vi "子VI-查看某框-不显示界面.vi"(0 "框号":dbl format="%#_13g", 1 "框组":T3(array[cluster]), 2 "计入缺陷的Z值阈值":i32 caption="值", 3 "临界Z值":i32, 4 "计入缺陷的面积阈值":i32, 5 "临界面积百分比值":dbl, 6 "图像Y向分辨率（mm/像素）":dbl, 7 "缺陷灰度阈值":dbl caption="值", 8 "?":T2(plugin-control), 9 "部位信息":string[](array[string])=["", "34.500000", "32.500000", "1121", "34", "54.955926", "分层类", "不合格", ""], 10 "判定为筋条的长宽比阈值":i32, 11 "图像X向分辨率（mm/像素）":dbl) -> (20 "全部检测结果":string[][](table), 25 "flag标记簇":cluster{"框号":dbl, "数值":i32})   [LabVIEW 2018]
uses:
  <vilib>/vision/NI_Vision_Development_Module.lvlib
panel:
  out "中心Y":dbl
  out "中心X":dbl
  in  "Tab Control":T1
  out "Threshold Image":T2(plugin-control)
  out "分层缺陷个数":i32
  out "合格？ 弥散类":string="fencengThreshold"
  out "合格？分层类":string="fencengThreshold"
  out "面积 (pixels)":i32
  in  "格式字符串 2":string="%f"
  in  "分隔符（'\\'代码显示）":string="\t"
  out "分层测量结果":i16[][](array[numeric])
  # "所选区域信息"
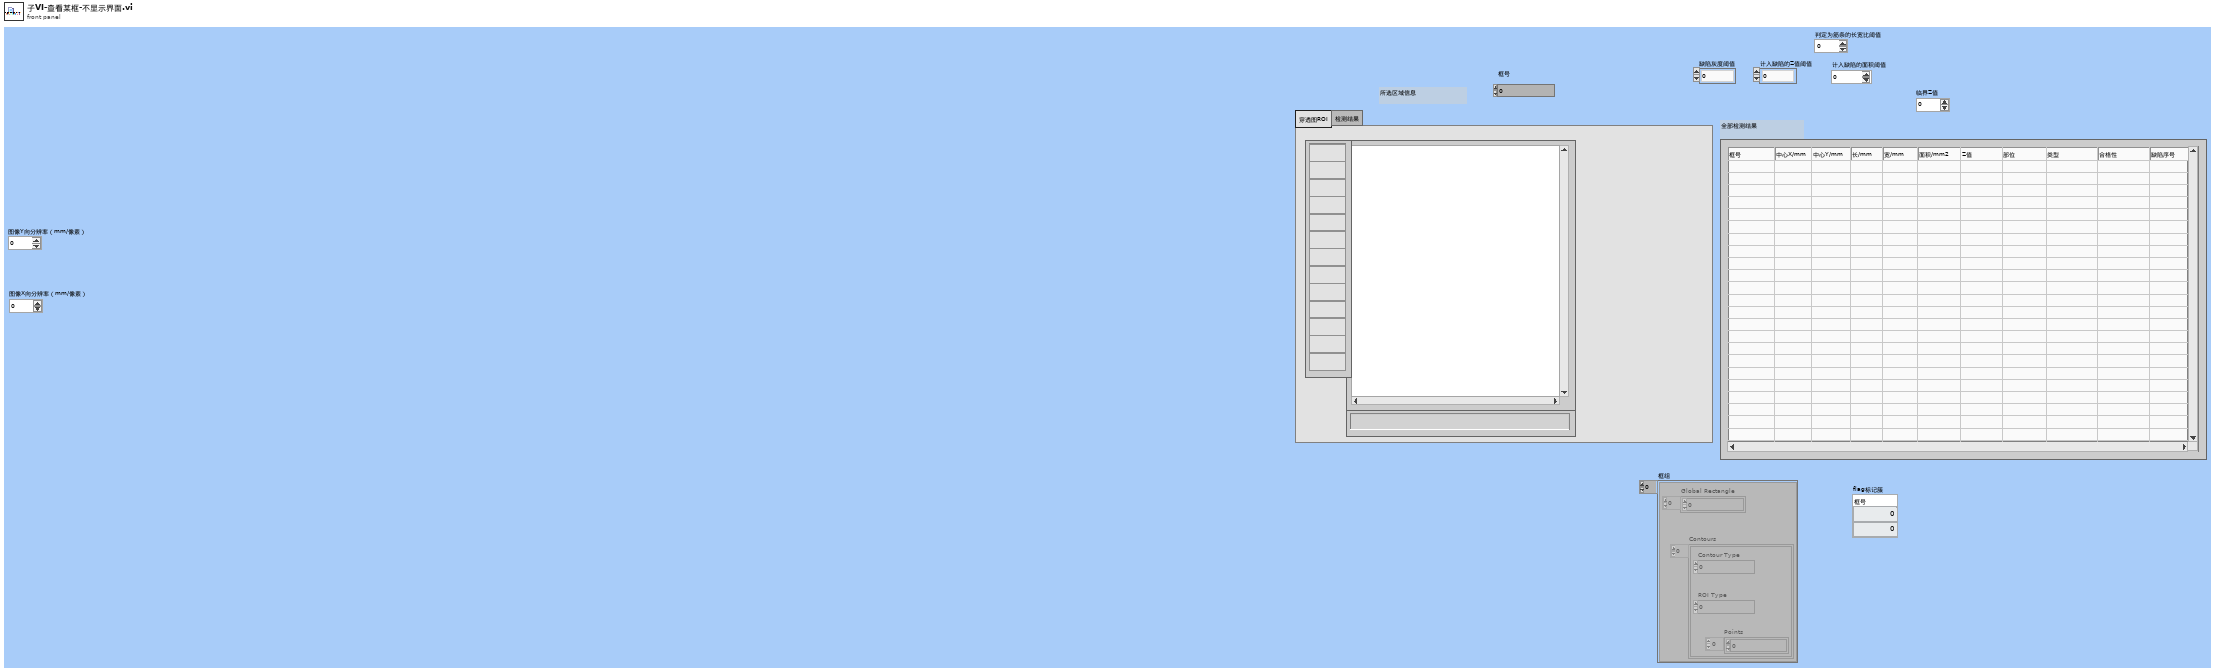
[diagram p1: front panel]
types:
  T1 = typedef "控件2.ctl" = enum32{"穿透图ROI", "检测结果"}
  T2 = typedef "IMAQ Image.ctl" = refnum<image>
  T3 = cluster{"Global Rectangle":i32[], "Contours":cluster{"Contour Type":u32, "ROI Type":u32, "Points":i32[]}[]}[]
  T4 = typedef "Image Type" = u32
  T5 = cluster{"Global Rectangle":i32[], "Contours":cluster{"Contour Type":u32, "ROI Type":u32, "Points":i32[]}[]}
  T6 = cluster{"Desired Font (Application)":enum16{"User-specified Font", "Application Font", "System Font", "Dialog Font"}, "[User-specified Font]":cluster{"Font Name":string, "Size":i16, "Strikeout?":bool, "Italic?":bool, "Underline?":bool, "Outline?":bool, "Shadow?":bool, "Bold?":bool, "Rotation Angle":dbl}, "Horizontal Alignment":i16, "Vertical Alignment":i16}
  T7 = cluster{"histogram":u32[], "Minimal Value":sgl, "Maximal Value":sgl, "Starting Value":sgl, "Interval Width":sgl, "Mean Value":sgl, "Standard  Variation":sgl, "Area (pixels)":i32}
  T8 = typedef "Particle Parameters" = i32
  T9 = cluster{"Area":dbl, "Number of Holes":dbl, "Bounding Rect":cluster{"Left":dbl, "Top":dbl, "Right":dbl, "Bottom":dbl}, "Center of Mass":cluster{"X":dbl, "Y":dbl}, "Orientation":dbl, "Dimensions":cluster{"Width":dbl, "Height":dbl}}[]
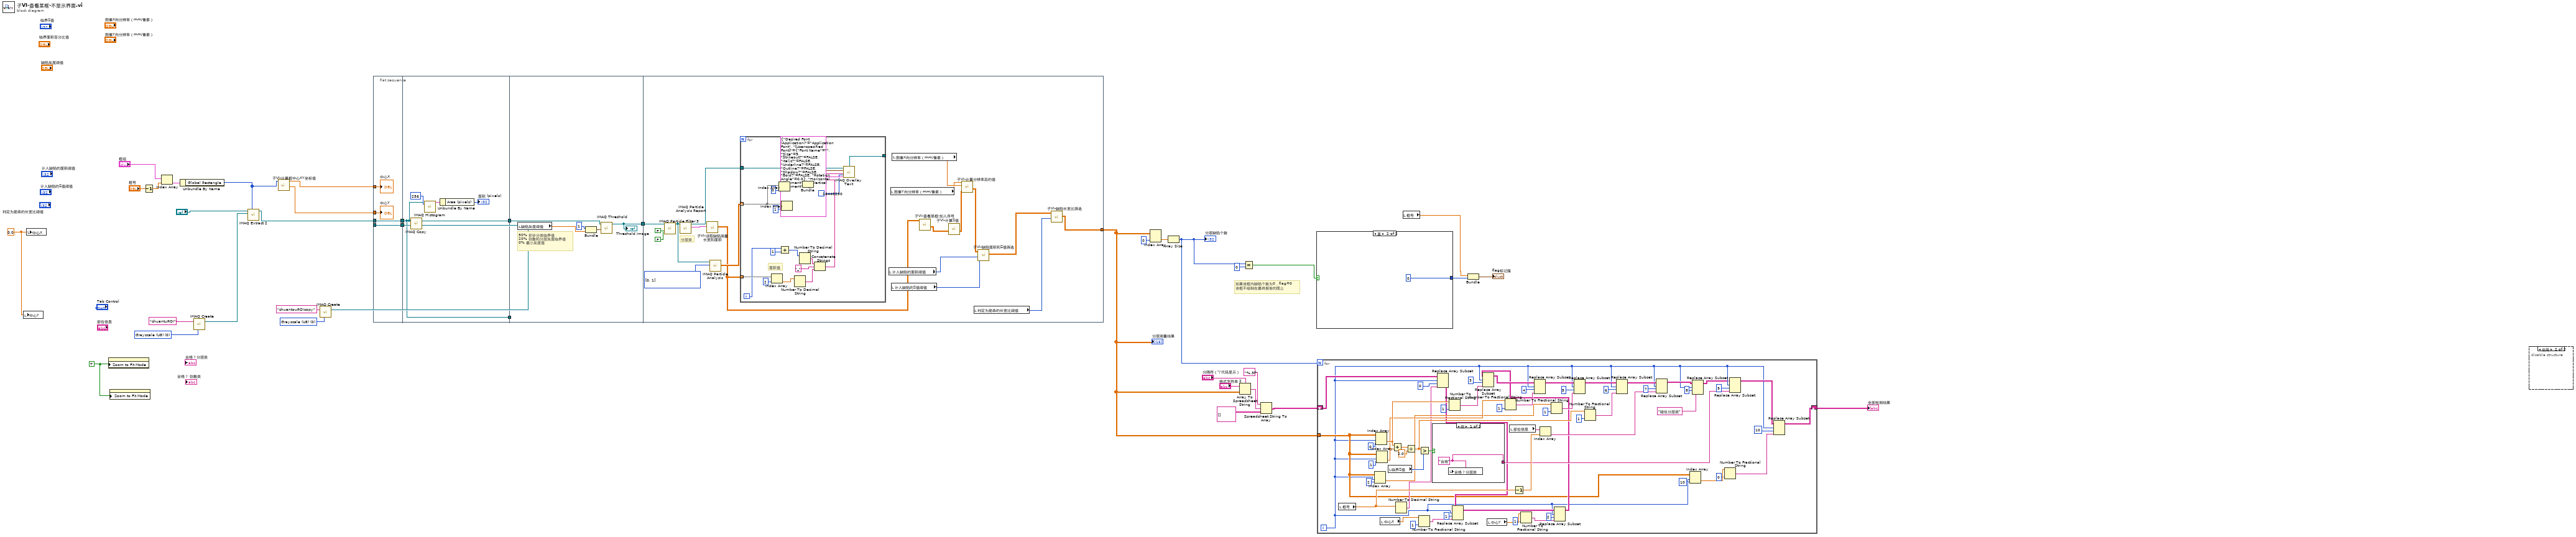
[diagram p0: block diagram]
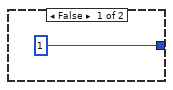
[diagram p2: hidden frame]
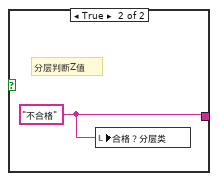
[diagram p3: hidden frame]
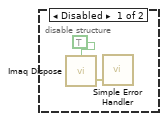
[diagram p4: hidden frame]
diagram:
  w10 = 0.0 ("中心X")
  w14 = T4 0 items=["Grayscale (U8)", "Grayscale (I16)", "Grayscale (SGL)", "Complex (CSG)", "RGB (U32)", "HSL (U32)", "RGB (U64)", "Grayscale (U16)"] ("Image Type")
  w19 = TRUE ("Zoom to Fit Mode")
  w33 = T4 0 items=["Grayscale (U8)", "Grayscale (I16)", "Grayscale (SGL)", "Complex (CSG)", "RGB (U32)", "HSL (U32)", "RGB (U64)", "Grayscale (U16)"] ("Image Type")
  # "如果该框内缺陷个数为0，flag=0\n该框不绘制在最终报告的图上"
  n1 = local write "中心Y"(w10) -> ()
  n2 = local write "中心X"(w10) -> ()
  n3 = property class="ImageControl"("Zoom to Fit Mode"=w19) -> ()  [unwired: 2 in, 2 out]
  n4 = property class="ImageControl"("Zoom to Fit Mode"=w19) -> ()  [unwired: 2 in, 2 out]
  n5 = Decrement(x="框号") -> (x-1=w35:dbl)
  n6 = Index Array(array="框组", index=w35) -> (element=w36:T5)
  n7 = Unbundle By Name(w36) -> ("Global Rectangle"=w13:i32[])
  n8 = call "IMAQ Create"("Image Name"="chuantuROI", "Image Type"=w33) -> ("New Image"=w32:T2)  [unwired: 3 in, 1 out]
  n9 = call "IMAQ Extract 2"("Optional Rectangle"=w13, "Image Dst"=w32, "Image Src"="?") -> ("Image Dst Out"=w7:T2)  [unwired: 7 in, 1 out]
  n10 = call "子VI-计算框中心XY坐标值.vi"("Global Rectangle"=w13) -> ("中心Y"=w11:dbl, "中心X"=w12:dbl)  [unwired: 9 in]
  n11 = call "IMAQ Create"("Image Name"="chuantouROIcopy", "Image Type"=w14) -> ("New Image"=w17:T2)  [unwired: 3 in, 1 out]
  n12 = flat-sequence {
    tunnel: w7 -> [w42]
    tunnel: [w42] -> w20
    tunnel: w17 -> [w41]
    tunnel: [w41] -> w16
    tunnel: w12 -> [w40]
    tunnel: w11 -> [w39]
    tunnel: [w45] -> w21
    tunnel: w20 -> [w45]
    tunnel: [w44] -> w18
    tunnel: w16 -> [w43]
    tunnel: [w53] -> w29
    tunnel: w21 -> [_]
    tunnel: w18 -> [w52]
    tunnel: [w67] -> w23
    tunnel: w29 -> [w70]
    frame #0 {
      "中心X" <- w40
      "中心Y" <- w39
    }
    frame #1 {
      n13 = call "IMAQ Copy"("Image Dst"=w43, "Image Src"=w45) -> ("Image Dst Out"=w44:T2)  [unwired: 4 in, 1 out]
      n14 = call "IMAQ Histogram"("Number of Classes"=256, "Image"=w45) -> ("Histogram Report"=w47:T7)  [unwired: 8 in, 1 out]
      n15 = Unbundle By Name(w47) -> ("Area (pixels)"=→"面积 (pixels)":i32)
    }
    frame #2 {
      # "50% 初步分类临界值\n20% 弥散和分层灰度临界值\n0% 最小灰度值"
      n16 = local read "缺陷灰度阈值"() -> (w50:dbl)
      n17 = Bundle(1, "缺陷灰度阈值"=w50) -> (w49:cluster{i32, "缺陷灰度阈值":dbl})  [unwired: 1 in]
      n18 = call "IMAQ Threshold"("Range"=w49, "Image Src"=w52) -> ("Image Dst Out"=w53:T2)  [unwired: 4 in, 5 out]
      "Threshold Image" <- w53
    }
    frame #3 {
      w63 = T8[] [0, 1] items=["Center of Mass X", "Center of Mass Y", "First Pixel X", "First Pixel Y", "Bounding Rect Left", "Bounding Rect Top", "Bounding Rect Right", "Bounding Rect Bottom", "Max Feret Diameter Start X", "Max Feret Diameter Start Y", "Max Feret Diameter End X", "Max Feret Diameter End Y", "Max Horiz. Segment Length Left", "Max Horiz. Segment Length Right", "Max Horiz. Segment Length Row", "-", "Bounding Rect Width", "Bounding Rect Height", "Bounding Rect Diagonal", "Perimeter", "Convex Hull Perimeter", "Holes' Perimeter", "Max Feret Diameter", "Equivalent Ellipse Major Axis", "Equivalent Ellipse Minor Axis", "Equivalent Ellipse Minor Axis (Feret)", "Equivalent Rect Long Side", "Equivalent Rect Short Side", "Equivalent Rect Diagonal", "Equivalent Rect Short Side (Feret)", "Average Horiz. Segment Length", "Average Vert. Segment Length", "Hydraulic Radius", "Waddel Disk Diameter", "-", "Area", "Holes' Area", "Particle & Holes' Area", "Convex Hull Area", "Image Area", "-", "Number of Holes", "Number of Horiz. Segments", "Number of Vert. Segments", "-", "Orientation", "Max Feret Diameter Orientation", "-", "% Area/Image Area", "% Area/(Particle & Holes' Area)", "Ratio of Equivalent Ellipse Axes", "Ratio of Equivalent Rect Sides", "-", "Elongation Factor", "Compactness Factor", "Heywood Circularity Factor", "Type Factor", "-", "Sum X", "Sum Y", "Sum XX", "Sum XY", "Sum YY", "Sum XXX", "Sum XXY", "Sum XYY", "Sum YYY", "-", "Moment of Inertia XX", "Moment of Inertia XY", "Moment of Inertia YY", "Moment of Inertia XXX", "Moment of Inertia XXY", "Moment of Inertia XYY", "Moment of Inertia YYY", "Norm. Moment of Inertia XX", "Norm. Moment of Inertia XY", "Norm. Moment of Inertia YY", "Norm. Moment of Inertia XXX", "Norm. Moment of Inertia XXY", "Norm. Moment of Inertia XYY", "Norm. Moment of Inertia YYY", "Hu Moment 1", "Hu Moment 2", "Hu Moment 3", "Hu Moment 4", "Hu Moment 5", "Hu Moment 6", "Hu Moment 7"] ("Pixel Measurements")
      # "分层类"
      n19 = call "IMAQ Particle Filter 3"("Image Src"=w70, "Keep/Remove Particles (F)"=FALSE, "Reject Border? (F)"=FALSE) -> ("Image Dst Out"=w62:T2)  [unwired: 10 in, 2 out]
      n20 = call "IMAQ Particle Analysis Report"("Image"=w62) -> ("Particle Reports (Pixels)"=w69:T9, "Image Out (duplicate)"=w60:T2)  [unwired: 5 in, 4 out]
      n21 = call "子VI-读取缺陷测量长宽和面积.vi"("Particle Reports (Pixels)"=w69) -> ("测量结果"=w59:dbl[][])  [unwired: 10 in]
      n22 = call "IMAQ Particle Analysis"("Pixel Measurements"=w63, "Image"=w62) -> ("Particle Measurements (Pixels)"=w61:dbl[][])  [unwired: 4 in, 5 out]
      n23 = for {
        tunnel: [w84] -> _
        tunnel: w60 -> [w92]
        tunnel: w61 -> [w89] mode=indexing
        tunnel: w59 -> [w80] mode=indexing
        i -> [w75]
        # "面积值"
        n24 = Index Array(array=w80, index=2 ("索引")) -> (element=w87:dbl)
        n25 = Index Array(array=w89, index=0 ("索引")) -> (element=w83:dbl)
        n26 = Add(x=w75, y=1) -> (x+y=w73:i32)
        n27 = Index Array(array=w89, index=1 ("索引")) -> (element=w82:dbl)
        n28 = Number To Decimal String(number=w87) -> (decimal integer string=w77:string)  [unwired: 1 in]
        n29 = Number To Decimal String(number=w73) -> (decimal integer string=w79:string)  [unwired: 1 in]
        n30 = Bundle("Numeric"=w83, "Numeric"=w82) -> (w81:cluster{"Numeric":dbl, "Numeric":dbl})  [unwired: 1 in]
        n31 = Concatenate Strings(w79, "_" ("字符串"), w77) -> (w78:string)
        n32 = call "IMAQ Overlay Text"("Text Color (black)"=u32 16448250, "Font, Size & Style"=T6 {"Desired Font (Application)"=enum."Application Font", "[User-specified Font]"={"Font Name"="", "Size"=9, "Strikeout?"=FALSE, "Italic?"=FALSE, "Underline?"=FALSE, "Outline?"=FALSE, "Shadow?"=FALSE, "Bold?"=FALSE, "Rotation Angle"=0.0}, "Horizontal Alignment"=0, "Vertical Alignment"=0}, "String"=w78, "Origin"=w81, "Image"=w92) -> ("Image Out"=w84:T2)  [unwired: 5 in, 1 out]
      }
      n33 = local read "计入缺陷的面积阈值"() -> (w68:i32)
      n34 = local read "图像Y向分辨率（mm/像素）"() -> (w64:dbl)
      n35 = local read "计入缺陷的Z值阈值"() -> (w58:i32)
      n36 = local read "图像X向分辨率（mm/像素）"() -> (w65:dbl)
      n37 = call "子VI-查看某框-加入序号.vi"("测量结果"=w59) -> ("测量结果 3"=w57:dbl[][])  [unwired: 9 in]
      n38 = call "子VI-计算Z值.vi"("分层测量结果"=w57) -> ("初始化的数组"=w56:dbl[][])  [unwired: 9 in]
      n39 = call "子VI-计算分辨率后的值.vi"("测量结果"=w56, "图像X向分辨率（mm/像素）"=w65, "图像Y向分辨率（mm/像素）"=w64) -> ("初始化的数组"=w55:dbl[][])  [unwired: 7 in]
      n40 = local read "判定为筋条的长宽比阈值"() -> (w66:i32)
      n41 = call "子VI-缺陷面积和Z值筛选.vi"("计入缺陷的Z值阈值"=w58, "计入分层缺陷的面积阈值"=w68, "分层测量结果"=w55) -> ("初始化的数组"=w54:dbl[][])  [unwired: 7 in, 1 out]
      n42 = call "子VI-缺陷长宽比筛选.vi"("判定为筋条的长宽比阈值"=w66, "分层测量结果"=w54) -> ("初始化的数组"=w67:dbl[][])  [unwired: 9 in]
    }
  }
  n43 = Index Array(array=w23, index (col)=0 ("禁用的索引 (列)")) -> (element=w31:dbl[])  [unwired: 1 in]
  n44 = Array Size(array=w31) -> (size(s)=w6:i32)
  "分层缺陷个数" <- w6
  n45 = Array To Spreadsheet String(delimiter (Tab)="分隔符（'\\'代码显示）", array=w23, 3:"格式字符串 2") -> (spreadsheet string=w26:string)
  n46 = Equal?(x=w6, y=0) -> (x = y?=w4:bool)
  n47 = Spreadsheet String To Array(format string="%.3f", spreadsheet string=w26, array type (2D Dbl)=string[][] [] ("Array")) -> (array=w22:string[][])  [unwired: 1 in]
  n48 = case shown="真" w4 {
    tunnel: [1 0] -> w2
    frame False {
    }
    frame True {
    }
  }
  n49 = for {
    N: w6 -> [_]
    tunnel: w23 -> [w101]
    shift-right: [w105] -> w9
    shift-left: w22 -> [w139]
    i -> [w98]
    n50 = local read "框号"() -> (w146:dbl)
    n51 = Index Array(array=w101, index (row)=w98, index (col)=2 ("索引 (列)")) -> (element=w124:dbl)
    n52 = Index Array(array=w101, index (row)=w98, index (col)=0 ("禁用的索引 (列)")) -> (element=w131:dbl)
    n53 = Index Array(array=w101, index (row)=w98, index (col)=1 ("禁用的索引 (列)")) -> (element=w130:dbl)
    n54 = local read "中心X"() -> (w121:dbl)
    n55 = local read "临界Z值"() -> (w153:i32)
    n56 = Add(x=w131, y=w130) -> (x+y=w154:dbl)
    n57 = Number To Decimal String(number=w146) -> (decimal integer string=w123:string)  [unwired: 1 in]
    n58 = Divide(x=w154, y=2.0) -> (x/y=w128:dbl)
    n59 = Number To Fractional String(number=w121, precision (6)=i16 1 ("精度(6)")) -> (F-format string=w120:string)  [unwired: 2 in]
    n60 = Greater?(x=w128, y=w153) -> (0:w155:bool)
    n61 = case shown="假" w155 {
      tunnel: [w156 w157] -> w126
      frame False {
        w156 = "合格" ("合格？")
        n62 = local write "合格？分层类"(w156) -> ()
      }
      frame True {
        w157 = "不合格" ("合格？")
        # "分层判断Z值"
        n63 = local write "合格？分层类"(w157) -> ()
      }
    }
    n64 = Replace Array Subset(array=w139, new element=w123, index (row)=w98, index (col)=0 ("索引 (列)")) -> (w113:string[][])
    n65 = Number To Fractional String(number=w131, precision (6)=i16 1 ("精度(6)")) -> (F-format string=w138:string)  [unwired: 2 in]
    n66 = Replace Array Subset(array=w113, new element=w120, index (row)=w98, index (col)=1 ("索引 (列)")) -> (w114:string[][])
    n67 = local read "中心Y"() -> (w118:dbl)
    n68 = Number To Fractional String(number=w130, precision (6)=i16 1 ("精度(6)")) -> (F-format string=w137:string)  [unwired: 2 in]
    n69 = local read "部位信息"() -> (w149:string[])
    n70 = Decrement(x=w146) -> (x-1=w148:dbl)
    n71 = Number To Fractional String(number=w118, precision (6)=i16 1 ("精度(6)")) -> (F-format string=w116:string)  [unwired: 2 in]
    n72 = Index Array(array=w149, index=w148) -> (element=w127:string)
    n73 = Number To Fractional String(number=w124, precision (6)=i16 1 ("精度(6)")) -> (F-format string=w134:string)  [unwired: 2 in]
    n74 = Replace Array Subset(array=w114, new element=w116, index (row)=w98, index (col)=2 ("索引 (列)")) -> (w112:string[][])
    n75 = Replace Array Subset(array=w112, new element=w138, index (row)=w98, index (col)=3 ("索引 (列)")) -> (w136:string[][])
    n76 = Replace Array Subset(array=w136, new element=w137, index (row)=w98, index (col)=4 ("索引 (列)")) -> (w135:string[][])
    n77 = Replace Array Subset(array=w135, new element=w134, index (row)=w98, index (col)=5 ("索引 (列)")) -> (w133:string[][])
    n78 = Number To Fractional String(number=w128, precision (6)=i16 1 ("精度(6)")) -> (F-format string=w129:string)  [unwired: 2 in]
    n79 = Replace Array Subset(array=w133, new element=w129, index (row)=w98, index (col)=6 ("索引 (列)")) -> (w132:string[][])
    n80 = Replace Array Subset(array=w132, new element=w127, index (row)=w98, index (col)=7 ("索引 (列)")) -> (w99:string[][])
    n81 = Index Array(array=w101, index (row)=w98, index (col)=10 ("索引 (列)")) -> (element=w103:dbl)
    n82 = Replace Array Subset(array=w99, new element="疑似分层类" ("新元素/子数组"), index (row)=w98, index (col)=8 ("禁用的索引 (列)")) -> (w95:string[][])
    n83 = Number To Fractional String(number=w103, precision (6)=i16 0 ("精度(6)")) -> (F-format string=w100:string)  [unwired: 2 in]
    n84 = Replace Array Subset(array=w95, new element=w126, index (row)=w98, index (col)=9 ("索引 (列)")) -> (w106:string[][])
    n85 = Replace Array Subset(array=w106, new element=w100, index (row)=w98, index (col)=10 ("禁用的索引 (列)")) -> (w105:string[][])
  }
  "全部检测结果" <- w9
  n86 = local read "框号"() -> (w3:dbl)
  n87 = Bundle("框号"=w3, w2) -> (→"flag标记簇":cluster{"框号":dbl, i32})  [unwired: 1 in]
  n88 = disable-structure shown="启用" {
    frame Disabled {
      n89 = call "Imaq Dispose"("All Images? (No)"=TRUE) -> ("error out"=w159:errorcluster)  [unwired: 5 in]
      n90 = call <vilib>:"Simple Error Handler.vi"("error in (no error)"=w159) -> ()  [unwired: 4 in, 5 out]
    }
    frame Enabled {
    }
  }
  "分层测量结果" <- w23
